vi "Stop Core.vi"(10 "final error code":i32, 11 "Digital Input in":refnum<class "Digital Input.lvclass">) -> (3 "Digital Input out":refnum<class "Digital Input.lvclass">)   [LabVIEW 2021, in "Digital Input.lvlib" / "Digital Input.lvclass"]
doc: "(<B>Filename</B>: Actor Framework.lvlib:Actor.lvclass:Stop Core.vi)\n\nDefines what the actor does before it stops. Use the <B>final error code</B> input to determine whether the actor shut down in response to an error.\n\nBy default, this method passes the Stop message along to all auto-stop nested actors. A descendant class may override this method to define additional behavior, such as shutting down any processes the actor initiated in its override of the Actor Core method."
uses:
  Digital Input.lvclass
  <vilib>/ActorFramework/Actor/Actor.lvclass
  Digital Input.lvclass/Digital Input.ctl
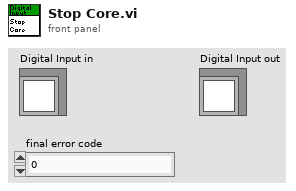
[diagram p1: front panel]
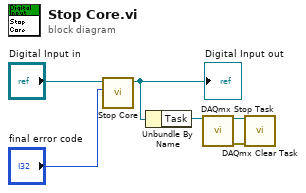
[diagram p0: block diagram]
diagram:
  n1 = call-parent "Stop Core.vi"("final error code"="final error code", "Actor in"="Digital Input in") -> ("Actor out"=w2:refnum<class "Digital Input.lvclass">)  [unwired: 9 in]
  "Digital Input out" <- w2
  n2 = Unbundle By Name(w2) -> ("Task"=w3:refnum<k21>)
  n3 = call <vilib>:"DAQmx Stop Task.vi"("task/channels in"=w3) -> ("task out"=w4:refnum<k21>, "error out"=w1:errorcluster)  [unwired: 13 in]
  n4 = call <vilib>:"DAQmx Clear Task.vi"("task in"=w4, "error in"=w1) -> ()  [unwired: 13 in, 1 out]
